vi "Setup EQE.vi"(6 "Skip cell?":bool, 8 "error in (no error)":errorcluster) -> (0 "error out":errorcluster)   [LabVIEW 2011]
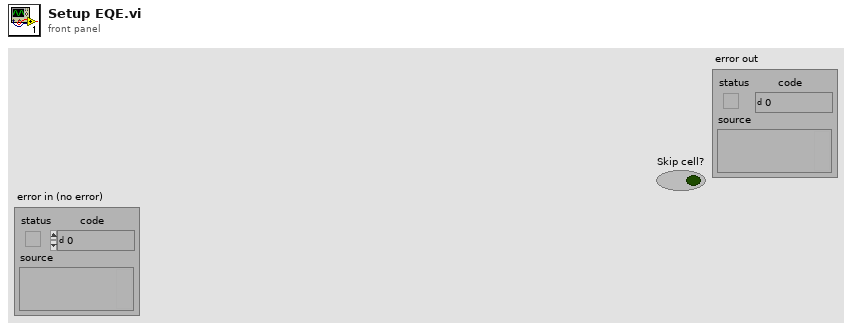
[diagram p1: front panel]
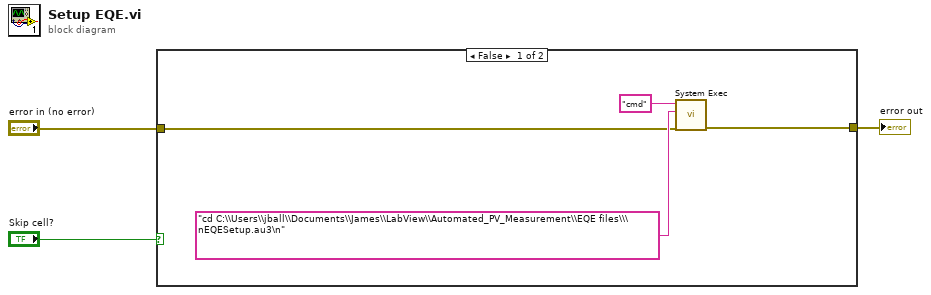
[diagram p0: block diagram]
diagram:
  n1 = case shown="False" "Skip cell?" {
    tunnel: [w5 w8] -> w2
    tunnel: "error in (no error)" -> [w4 w8]
    frame False {
      n2 = call <vilib>:"System Exec.vi"("error in (no error)"=w4, "standard input"="cd C:\\Users\\jball\\Documents\\James\\LabView\\Automated_PV_Measurement\\EQE files\\\nEQESetup.au3\n", "command line"="cmd") -> ("error out"=w5:errorcluster)  [unwired: 5 in, 3 out]
    }
    frame True {
    }
  }
  "error out" <- w2
